vi "Interactive Manager UI.vi"() -> ()   [LabVIEW 2021]
uses:
  CIFPluginManager/gRPC/CIF_Manager_client/RPC Messages/cif_manager_PluginConfig.ctl
  CIFUI/CIF_UI.lvclass/CIF_UI.ctl
  CIFPluginManager/gRPC/CIF_Manager_Client_Wrapper/CIFManagerClientWrapper.lvlib
  CIFUI/CIF_UI.lvclass
  CIFPluginManager/gRPC/CIF_Manager_client/CIF_Manager_client.lvlib
panel:
  in  "Reset Config":bool
  in  "Reset Info":bool
  in  "Get Config":bool
  out "Config":string
  in  "All Config":bool
  in  "Destroy":bool
  in  "Abort All Plugins":bool
  in  "Abort Plugin":bool
  in  "Reset Errors":bool
  in  "Get Info":bool
  in  "Get Errors":bool
  in  "Get Loaded Plugins":bool
  in  "Update Plugin Types":bool
  in  "Errors":i32(listbox)=-1
  in  "Loaded Plugins":string(tree)
  in  "plugin_name":string
  out "Info":string
  in  "All Info":bool
  in  "All Errors":bool
  in  "Plugin":T1
  in  "Load Plugin":bool
  out "final errror":errorcluster
  in  "Clear Error":bool
  in  "stop":bool
  in  "Plugin Types":string(tree)
  out "local error":errorcluster
  in  "address":string="192.168.1.160:15882"
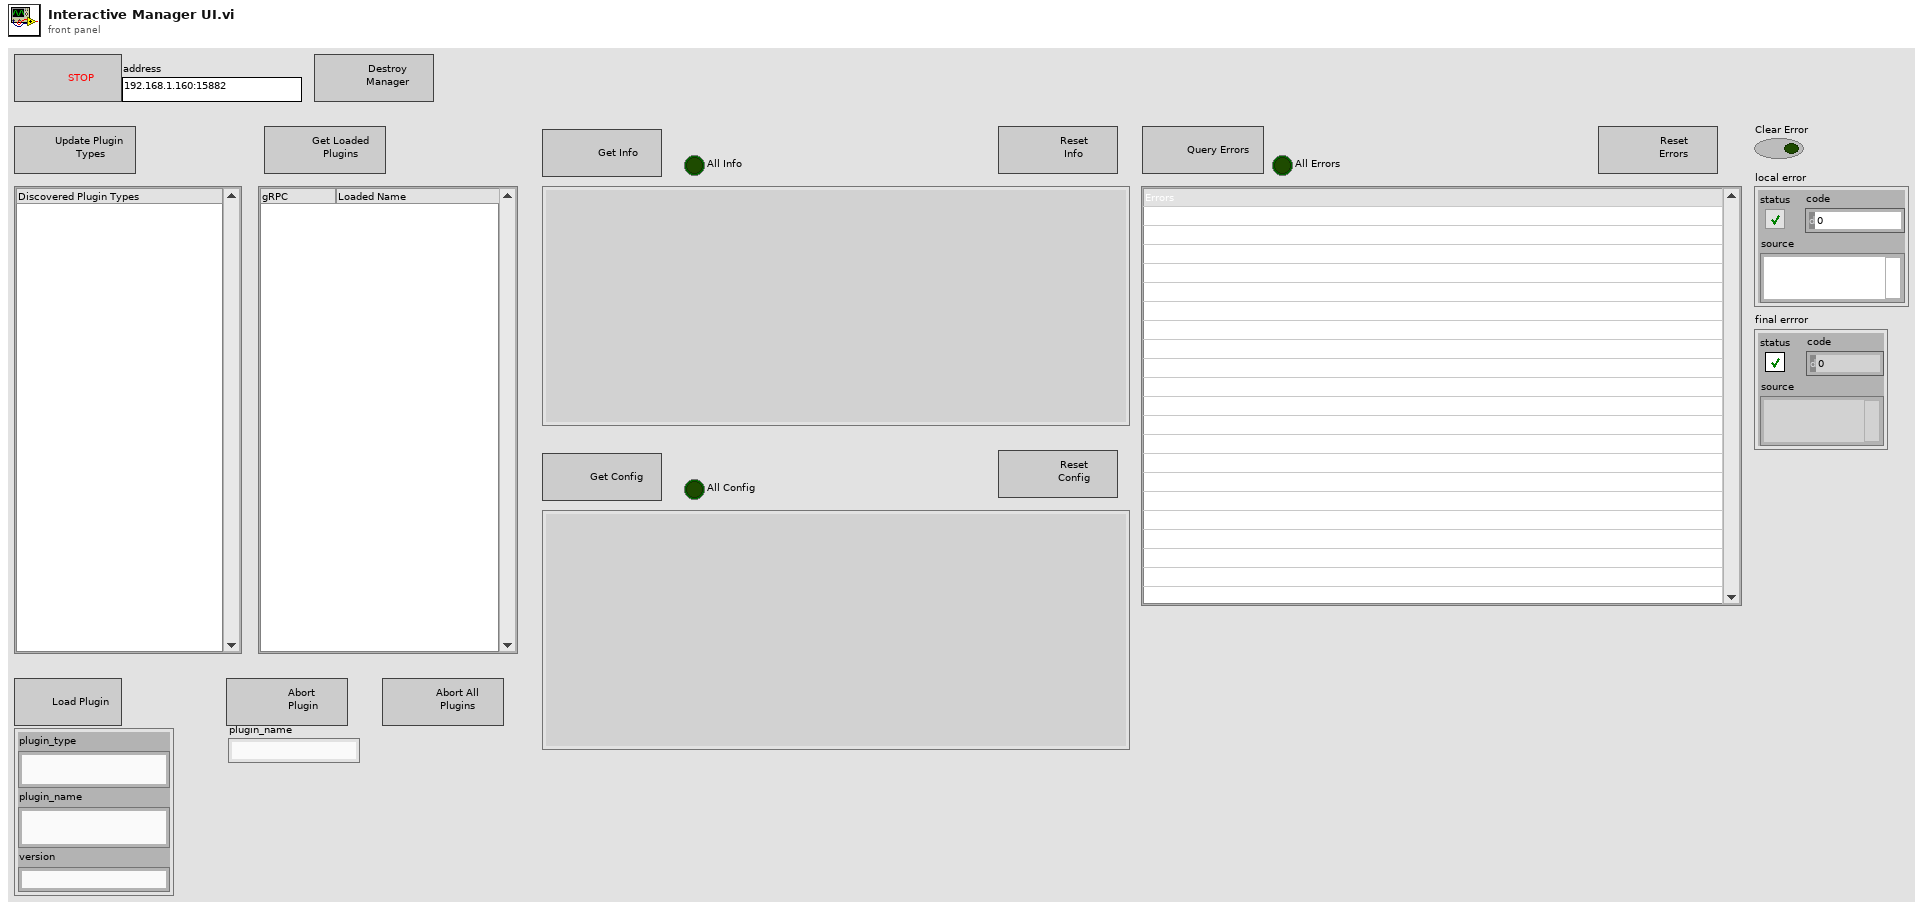
[diagram p1: front panel]
types:
  T1 = typedef "CIF_Manager_client.lvlib/cif_manager_PluginConfig.ctl" = cluster{"plugin_type":string, "plugin_name":string, "version":string}
  T2 = typedef "grpc-lvsupport-release.lvlib/grpcId.ctl" = u64
  T3 = typedef "CIF_Manager_client.lvlib/cif_manager_PluginType.ctl" = cluster{"plugin_type":string, "plugin_version":T4}
  T4 = typedef "CIF_Manager_client.lvlib/cif_manager_PluginVersion.ctl" = cluster{"major_version":i32, "minor_version":i32, "fix_version":i32, "build_version":i32}
  T5 = typedef "CIF_Manager_client.lvlib/cif_manager_PluginInfo.ctl" = cluster{"plugin_name":string, "plugin_type":string, "grpc_port":i32, "plugin_version":T4, "status":T6}
  T6 = typedef "CIF_Manager_client.lvlib/cif_plugincore_StatusData.ctl" = cluster{"state":T7, "timing_statistics":T8, "fifo_statistics":T10, "error":T11, "monitor_doubles":T12, "monitor_u64s":T13, "monitor_i64s":T14}
  T7 = typedef "CIF_Manager_client.lvlib/cif_plugincore_StatusData_State.ctl" = enum32{"NULL", "CREATING", "LISTENING", "RUNNING", "CLEANINGUP", "DESTROYING"}
  T8 = typedef "CIF_Manager_client.lvlib/cif_plugincore_TimingStatistics.ctl" = cluster{"period":T9, "wake_error":T9, "execute":T9, "housekeep":T9, "idle":T9}
  T9 = typedef "CIF_Manager_client.lvlib/cif_plugincore_TimingStatsBasic.ctl" = cluster{"max":i32, "min":i32}
  T10 = typedef "CIF_Manager_client.lvlib/cif_plugincore_FifoStatistics.ctl" = cluster{"from_t0":T9, "from_previous_plugin":T9, "output_error":T9}
  T11 = typedef "CIF_Manager_client.lvlib/cif_plugincore_Error.ctl" = cluster{"status":bool, "code":i32}
  T12 = typedef "CIF_Manager_client.lvlib/cif_plugincore_MonitorDoubles.ctl" = cluster{"double_1":dbl, "double_2":dbl, "double_3":dbl, "double_4":dbl}
  T13 = typedef "CIF_Manager_client.lvlib/cif_plugincore_MonitorU64.ctl" = cluster{"u64_1":u64, "u64_2":u64, "u64_3":u64, "u64_4":u64}
  T14 = typedef "CIF_Manager_client.lvlib/cif_plugincore_MonitorI64.ctl" = cluster{"i64_1":i64, "i64_2":i64, "i64_3":i64, "i64_4":i64}
  T15 = typedef "CIF_Manager_client.lvlib/cif_manager_ErrorInfo.ctl" = cluster{"error_status":bool, "error_code":i32, "plugin":string, "time":string, "message":string, "location":string}
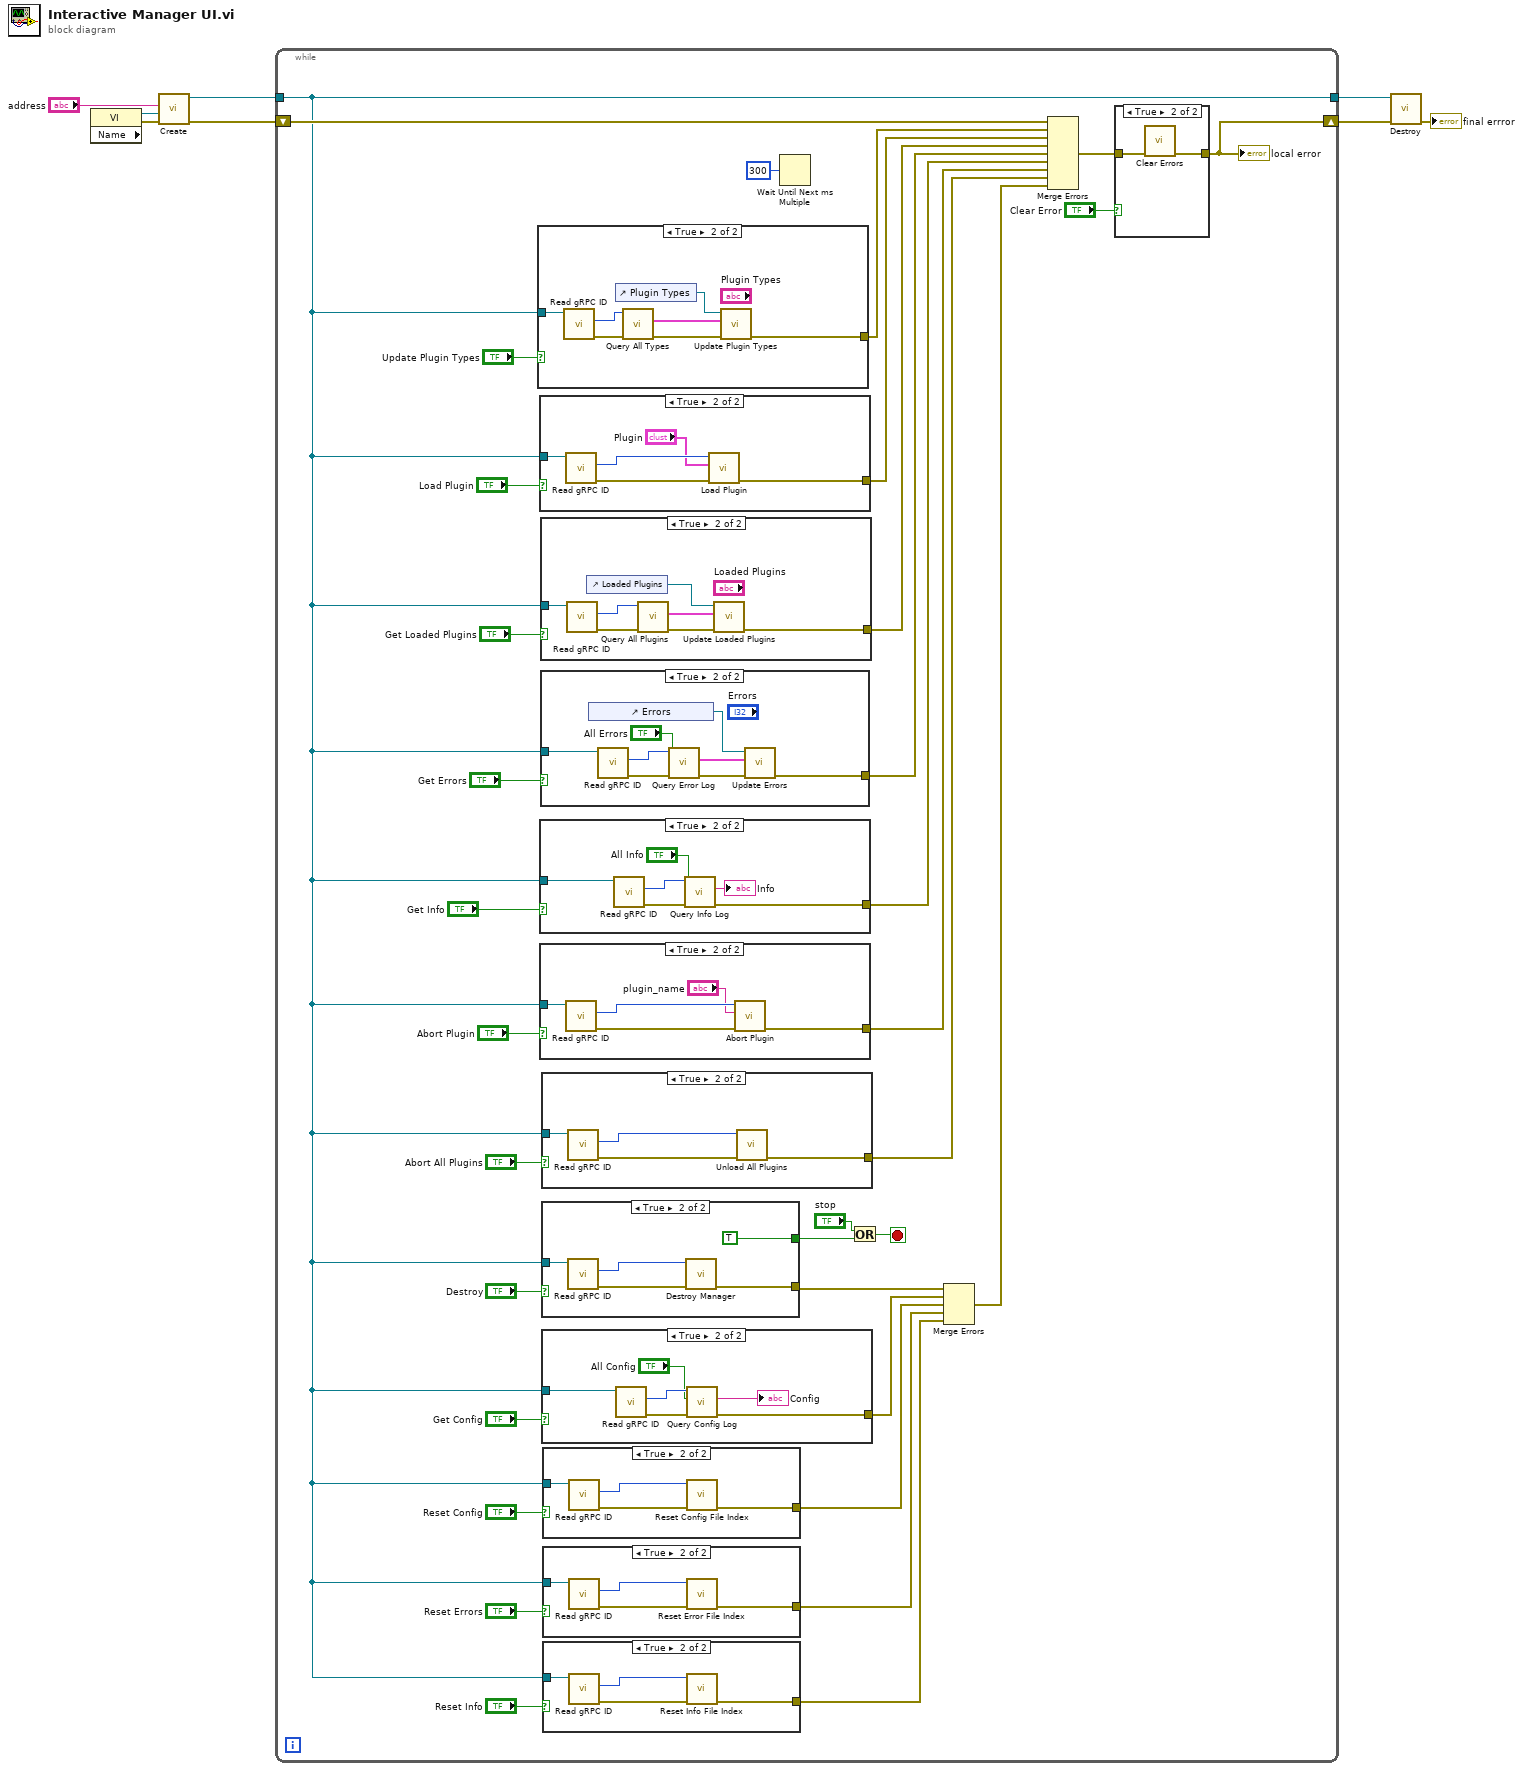
[diagram p0: block diagram]
diagram:
  n1 = property class="VI" props=["Name"]() -> (reference out=w6:refnum<vi>, error out=w7:errorcluster)  [unwired: 2 in, 1 out]
  n2 = call "Create.vi"("error in (no error)"=w7, "VI Reference"=w6, "Manager Address"="address") -> ("error out"=w4:errorcluster, "CIF_UI out"=w5:refnum<class "CIF_UI.lvclass">)  [unwired: 7 in]
  n3 = while {
    tunnel: w5 -> [w13]
    shift-right: [w38] -> w2
    shift-left: w4 -> [w42]
    tunnel: [w13] -> w3
    stop <- w21 stop-if-true
    n4 = case shown="True" "Update Plugin Types" {
      tunnel: w13 -> [_ w110]
      tunnel: [_ w104] -> w41
      frame False {
      }
      frame True {
        n5 = call "Read gRPC ID.vi"("CIF_UI in"=w110) -> ("error out"=w105:errorcluster, "gRPCid"=w106:T2)  [unwired: 8 in, 1 out]
        n6 = control-ref of="Plugin Types"() -> (w108:refnum<vi>)
        n7 = call "Query All Types.vi"("error in"=w105, "gRPC ID in"=w106) -> ("error out"=w109:errorcluster, "plugin_types"=w107:T3[])  [unwired: 7 in, 1 out]
        n8 = call "Update Plugin Types.vi"("error in (no error)"=w109, "plugin_types"=w107, "Plugin Types ref in"=w108) -> ("error out"=w104:errorcluster)  [unwired: 7 in, 1 out]
      }
    }
    n9 = case shown="True" "Load Plugin" {
      tunnel: w13 -> [_ w100]
      tunnel: [_ w97] -> w35
      frame False {
      }
      frame True {
        n10 = call "Read gRPC ID.vi"("CIF_UI in"=w100) -> ("error out"=w98:errorcluster, "gRPCid"=w99:T2)  [unwired: 8 in, 1 out]
        n11 = call "Load Plugin.vi"("error in"=w98, "Plugin"="Plugin", "gRPC ID in"=w99) -> ("error out"=w97:errorcluster)  [unwired: 7 in, 1 out]
      }
    }
    n12 = case shown="True" "Get Info" {
      tunnel: w13 -> [_ w80]
      tunnel: [_ w77] -> w32
      frame False {
      }
      frame True {
        n13 = call "Read gRPC ID.vi"("CIF_UI in"=w80) -> ("error out"=w78:errorcluster, "gRPCid"=w79:T2)  [unwired: 8 in, 1 out]
        n14 = call "Query Info Log.vi"("error in"=w78, "query_all"="All Info", "gRPC ID in"=w79) -> ("error out"=w77:errorcluster, "Info"=→"Info":string)  [unwired: 6 in, 1 out]
      }
    }
    n15 = case shown="True" "Abort Plugin" {
      tunnel: w13 -> [_ w74]
      tunnel: [_ w71] -> w31
      frame False {
      }
      frame True {
        n16 = call "Read gRPC ID.vi"("CIF_UI in"=w74) -> ("error out"=w72:errorcluster, "gRPCid"=w73:T2)  [unwired: 8 in, 1 out]
        n17 = call "Abort Plugin.vi"("error in"=w72, "plugin_name"="plugin_name", "gRPC ID in"=w73) -> ("error out"=w71:errorcluster)  [unwired: 7 in, 1 out]
      }
    }
    n18 = case shown="True" "Get Loaded Plugins" {
      tunnel: w13 -> [_ w95]
      tunnel: [_ w89] -> w34
      frame False {
      }
      frame True {
        n19 = call "Read gRPC ID.vi"("CIF_UI in"=w95) -> ("error out"=w93:errorcluster, "gRPCid"=w94:T2)  [unwired: 8 in, 1 out]
        n20 = control-ref of="Loaded Plugins"() -> (w90:refnum<vi>)
        n21 = call "Query All Plugins.vi"("error in"=w93, "gRPC ID in"=w94) -> ("error out"=w91:errorcluster, "plugin_info"=w92:T5[])  [unwired: 7 in, 1 out]
        n22 = call "Update Loaded Plugins.vi"("error in (no error)"=w91, "plugin_info"=w92, "Loaded Plugins ref in"=w90) -> ("error out"=w89:errorcluster)  [unwired: 7 in, 1 out]
      }
    }
    n23 = case shown="True" "Get Errors" {
      tunnel: w13 -> [_ w88]
      tunnel: [_ w81] -> w33
      frame False {
      }
      frame True {
        n24 = control-ref of="Errors"() -> (w82:refnum<vi>)
        n25 = call "Read gRPC ID.vi"("CIF_UI in"=w88) -> ("error out"=w86:errorcluster, "gRPCid"=w87:T2)  [unwired: 8 in, 1 out]
        n26 = call "Query Error Log.vi"("error in"=w86, "query_all"="All Errors", "gRPC ID in"=w87) -> ("error out"=w84:errorcluster, "error_info"=w83:T15[])  [unwired: 6 in, 1 out]
        n27 = call "Update Errors.vi"("error in (no error)"=w84, "error_info"=w83, "Error MCLB reference in"=w82) -> ("error out"=w81:errorcluster)  [unwired: 7 in, 1 out]
      }
    }
    n28 = case shown="True" "Abort All Plugins" {
      tunnel: w13 -> [_ w69]
      tunnel: [_ w66] -> w30
      frame False {
      }
      frame True {
        n29 = call "Read gRPC ID.vi"("CIF_UI in"=w69) -> ("error out"=w67:errorcluster, "gRPCid"=w68:T2)  [unwired: 8 in, 1 out]
        n30 = call "Unload All Plugins.vi"("error in"=w67, "gRPC ID in"=w68) -> ("error out"=w66:errorcluster)  [unwired: 8 in, 1 out]
      }
    }
    n31 = case shown="True" "Destroy" {
      tunnel: w13 -> [_ w65]
      tunnel: [_ w62] -> w18
      tunnel: [_ TRUE] -> w22
      frame False {
      }
      frame True {
        n32 = call "Read gRPC ID.vi"("CIF_UI in"=w65) -> ("error out"=w63:errorcluster, "gRPCid"=w64:T2)  [unwired: 8 in, 1 out]
        n33 = call "Destroy Manager.vi"("error in"=w63, "gRPC ID in"=w64) -> ("error out"=w62:errorcluster)  [unwired: 8 in, 1 out]
      }
    }
    n34 = case shown="True" "Get Config" {
      tunnel: w13 -> [_ w60]
      tunnel: [_ w57] -> w16
      frame False {
      }
      frame True {
        n35 = call "Read gRPC ID.vi"("CIF_UI in"=w60) -> ("error out"=w58:errorcluster, "gRPCid"=w59:T2)  [unwired: 8 in, 1 out]
        n36 = call "Query Config Log.vi"("error in"=w58, "query_all"="All Config", "gRPC ID in"=w59) -> ("error out"=w57:errorcluster, "Config"=→"Config":string)  [unwired: 6 in, 1 out]
      }
    }
    n37 = case shown="True" "Reset Config" {
      tunnel: w13 -> [_ w54]
      tunnel: [_ w51] -> w15
      frame False {
      }
      frame True {
        n38 = call "Read gRPC ID.vi"("CIF_UI in"=w54) -> ("error out"=w52:errorcluster, "gRPCid"=w53:T2)  [unwired: 8 in, 1 out]
        n39 = call "Reset Config File Index.vi"("error in"=w52, "gRPC ID in"=w53) -> ("error out"=w51:errorcluster)  [unwired: 8 in, 1 out]
      }
    }
    n40 = case shown="True" "Reset Errors" {
      tunnel: w13 -> [_ w50]
      tunnel: [_ w47] -> w10
      frame False {
      }
      frame True {
        n41 = call "Read gRPC ID.vi"("CIF_UI in"=w50) -> ("error out"=w48:errorcluster, "gRPCid"=w49:T2)  [unwired: 8 in, 1 out]
        n42 = call "Reset Error File Index.vi"("error in"=w48, "gRPC ID in"=w49) -> ("error out"=w47:errorcluster)  [unwired: 8 in, 1 out]
      }
    }
    n43 = case shown="True" "Reset Info" {
      tunnel: w13 -> [_ w46]
      tunnel: [_ w43] -> w9
      frame False {
      }
      frame True {
        n44 = call "Read gRPC ID.vi"("CIF_UI in"=w46) -> ("error out"=w44:errorcluster, "gRPCid"=w45:T2)  [unwired: 8 in, 1 out]
        n45 = call "Reset Info File Index.vi"("error in"=w44, "gRPC ID in"=w45) -> ("error out"=w43:errorcluster)  [unwired: 8 in, 1 out]
      }
    }
    n46 = Wait Until Next ms Multiple(millisecond multiple=u32 300) -> ()  [unwired: 1 out]
    n47 = Or(x="stop", y=w22) -> (x .or. y?=w21:bool)
    n48 = Merge Errors(w18, w16, w15, w10, w9) -> (w19:errorcluster)
    n49 = Merge Errors(w42, w41, w35, w34, w33, w32, w31, w30, w19) -> (w39:errorcluster)
    n50 = case shown="True" "Clear Error" {
      tunnel: w39 -> [w101 w103]
      tunnel: [w101 w102] -> w38
      frame False {
      }
      frame True {
        n51 = call <vilib>:"Clear Errors.vi"("error in (no error)"=w103) -> ("error out"=w102:errorcluster)  [unwired: 5 in, 1 out]
      }
    }
    "local error" <- w38
  }
  n52 = call "Destroy.vi"("error in (no error)"=w2, "CIF_UI in"=w3) -> ("error out"=→"final errror":errorcluster)  [unwired: 8 in, 1 out]
